vi "HTR_Check.vi"(1 "HTR_Fault ref":refnum<vi>, 4 "HTR ON Ref":refnum<vi>, 6 "Logging Ref":refnum<vi>, 8 "error in (no error)":errorcluster, 9 "HTR_Monitor Ref":refnum<vi>, 11 "Heater Test Options":T1 {"Heater Current Tolerance (%)" min=1.0 max=100.0; "Heater Nominal Current (A)" min=0.0 max=1.0}) -> (0 "error out":errorcluster)   [LabVIEW 2025]
uses:
  controls/HTR Test Options.ctl
  controls/TestFailOptions.ctl
  <vilib>/ErrorRing/Error Ring.xnode
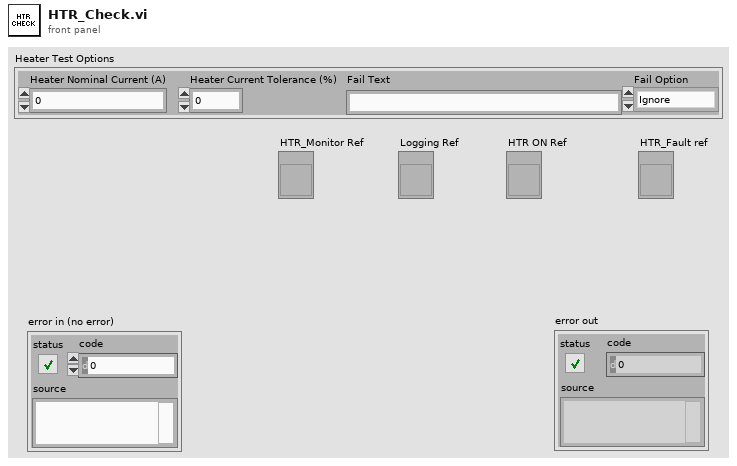
[diagram p1: front panel]
types:
  T1 = typedef "HTR Test Options.ctl" = cluster{"Heater Nominal Current (A)":dbl, "Heater Current Tolerance (%)":dbl, "Fail Text":string, "Fail Option":T2}
  T2 = typedef "TestFailOptions.ctl" = enum16{"Ignore", "Halt End Cycle", "Skip Rest Of Cycle"}
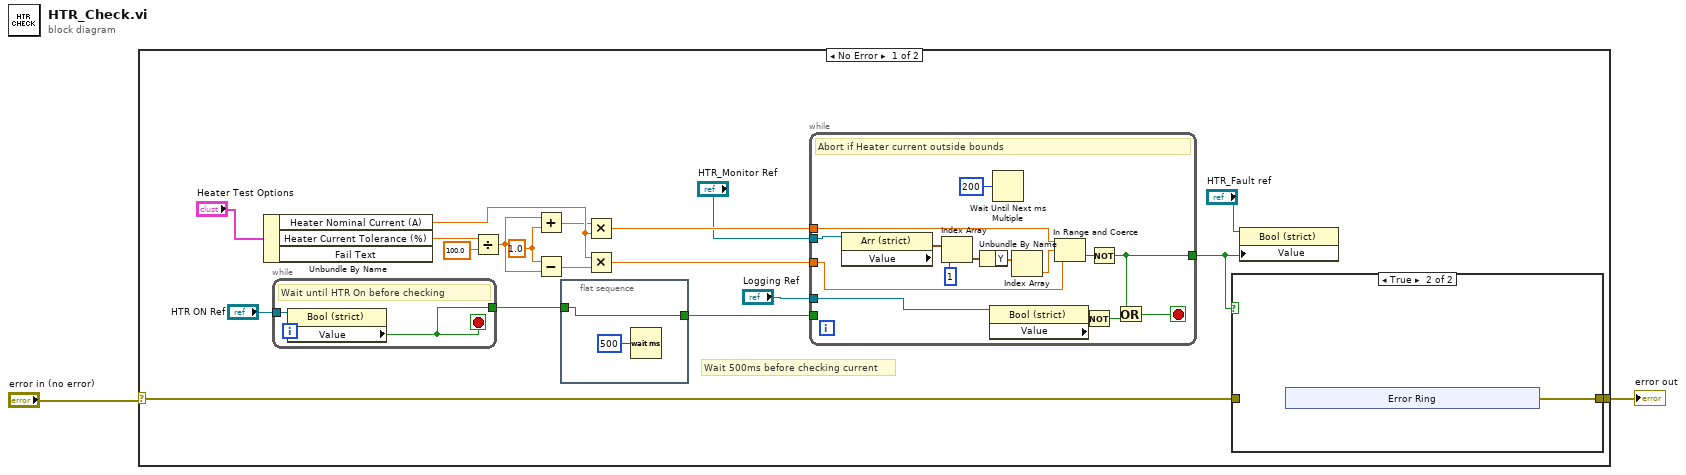
[diagram p0: block diagram]
diagram:
  n1 = case shown="No Error" "error in (no error)" {
    selector: "error in (no error)" -> [w6 w44]
    tunnel: [w5 w44] -> w1
    frame No Error {
      w14 = 1.0 ("x")
      # "Wait 500ms before checking current"
      n2 = Unbundle By Name("Heater Test Options") -> ("Heater Nominal Current (A)"=w18:dbl, "Heater Current Tolerance (%)"=w12:dbl)  [unwired: 1 out]
      n3 = while {
        tunnel: [w28] -> w4
        tunnel: "HTR ON Ref" -> [w27]
        stop <- w28 stop-if-true
        # "Wait until HTR On before checking"
        n4 = property class="Bool (strict)"(reference=w27) -> ("Value"=w28:bool)  [unwired: 1 in, 2 out]
      }
      n5 = Divide(x=w12, y=100.0) -> (x/y=w15:dbl)
      n6 = Add(x=w15, y=w14) -> (x+y=w16:dbl)
      n7 = Subtract(x=w14, y=w15) -> (x-y=w17:dbl)
      n8 = flat-sequence {
        tunnel: w4 -> [w22]
        tunnel: [w22] -> w3
        frame #0 {
          n9 = Wait (ms)(milliseconds to wait=u32 500) -> ()  [unwired: 1 out]
        }
      }
      n10 = Multiply(x=w16, y=w18) -> (x*y=w20:dbl)
      n11 = Multiply(x=w18, y=w17) -> (x*y=w21:dbl)
      n12 = while {
        tunnel: w20 -> [w38]
        tunnel: w21 -> [w37]
        tunnel: [w34] -> w7
        tunnel: "HTR_Monitor Ref" -> [w31]
        tunnel: "Logging Ref" -> [w30]
        tunnel: w3 -> [_]
        stop <- w33 stop-if-true
        # "Abort if Heater current outside bounds"
        n13 = property class="Arr (strict)"(reference=w31) -> ("Value"=w43:waveform(dbl)[])  [unwired: 1 in, 2 out]
        n14 = Index Array(array=w43, index=1) -> (element=w41:waveform(dbl))
        n15 = Unbundle By Name(w41) -> ("Y"=w40:dbl[])
        n16 = property class="Bool (strict)"(reference=w30) -> ("Value"=w35:bool)  [unwired: 1 in, 2 out]
        n17 = Wait Until Next ms Multiple(millisecond multiple=u32 200) -> ()  [unwired: 1 out]
        n18 = Index Array(array=w40) -> (element=w39:dbl)  [unwired: 1 in]
        n19 = In Range and Coerce(upper limit=w38, x=w39, lower limit=w37) -> (In Range?=w36:bool)  [unwired: 1 out]
        n20 = Not(x=w35) -> (.not. x?=w32:bool)
        n21 = Not(x=w36) -> (.not. x?=w34:bool)
        n22 = Or(x=w34, y=w32) -> (x .or. y?=w33:bool)
      }
      n23 = case shown="True" w7 {
        tunnel: w6 -> [w24 _]
        tunnel: [w24 w25] -> w5
        frame False {
        }
        frame True {
          n24 = xnode "Error Ring"() -> ("error out"=w25:errorcluster)
        }
      }
      n25 = property class="Bool (strict)"(reference="HTR_Fault ref", "Value"=w7) -> ()  [unwired: 1 in, 2 out]
    }
    frame Error {
    }
  }
  "error out" <- w1
